vi "DAQElevador.vi"() -> ()   [LabVIEW 2018]
uses:
  EstadoElevador.ctl
panel:
  out "Piso":u32
  out "PteH":i32
  out "Estado Actual":T1
  out "Boton":u32
  in  "stop":bool
  in  "Sensor 1":bool
  in  "Sensor 2":bool
  in  "Sensor 3":bool
  in  "Sensor 4":bool
  in  "Piso 4":bool
  in  "Piso 3":bool
  in  "Piso 2":bool
  in  "Piso 1":bool
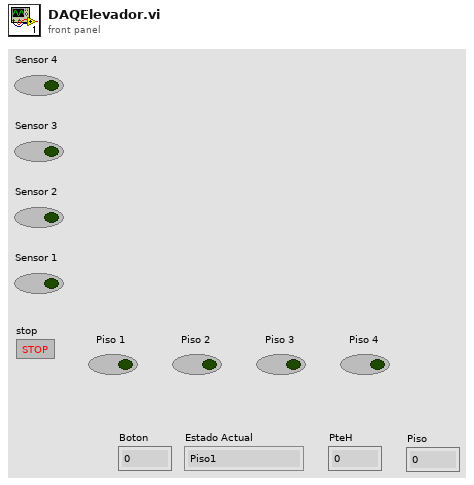
[diagram p1: front panel]
types:
  T1 = typedef "EstadoElevador.ctl" = enum16{"Piso1", "Piso2", "Piso3", "Piso4", "SubiendoPiso2", "SubiendoPiso3", "SubiendoPiso4", "BajandoPiso1", "BajandoPiso2", "BajandoPiso3"}
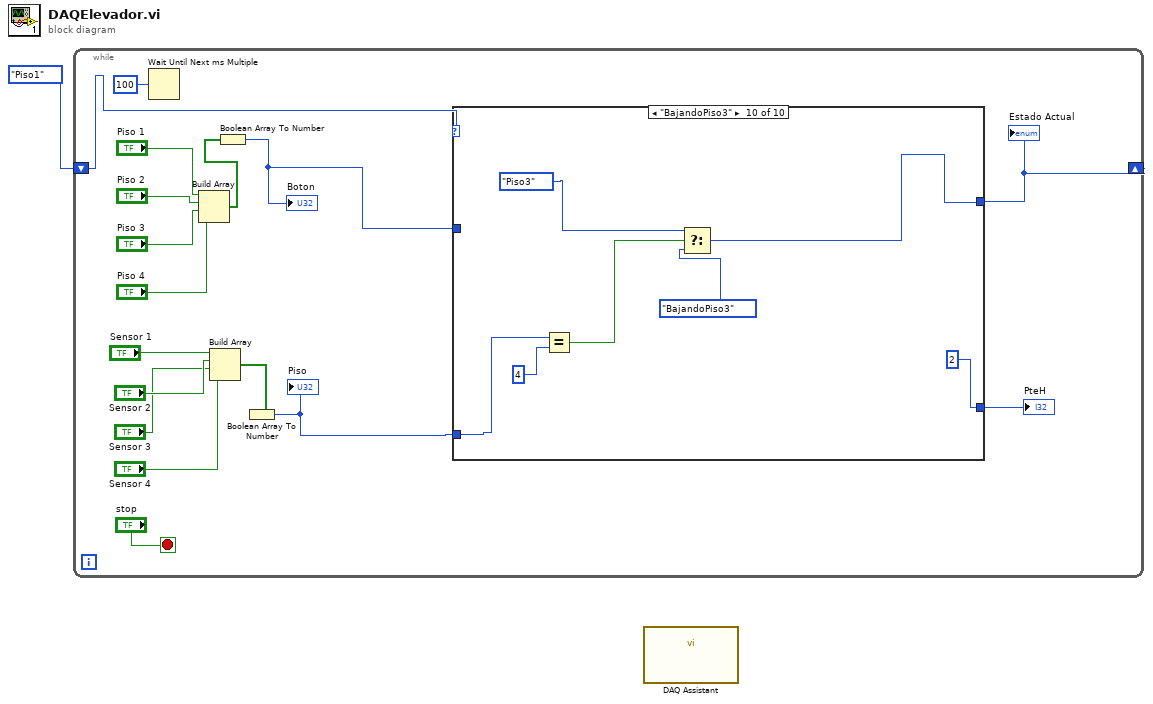
[diagram p0: block diagram]
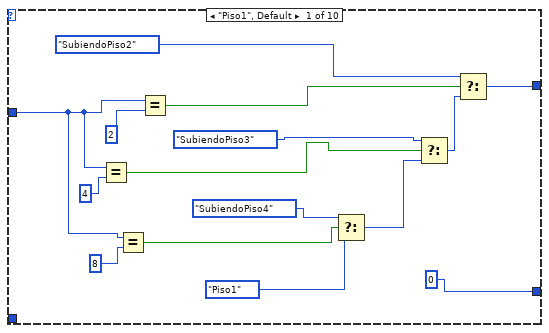
[diagram p2: hidden frame]
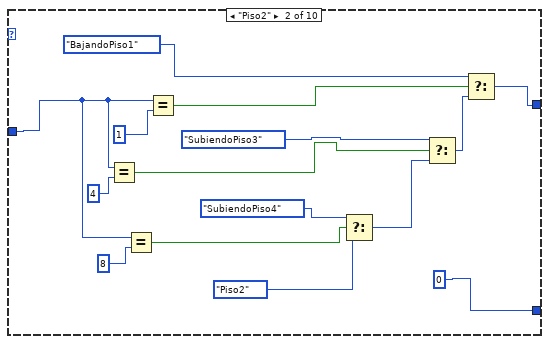
[diagram p3: hidden frame]
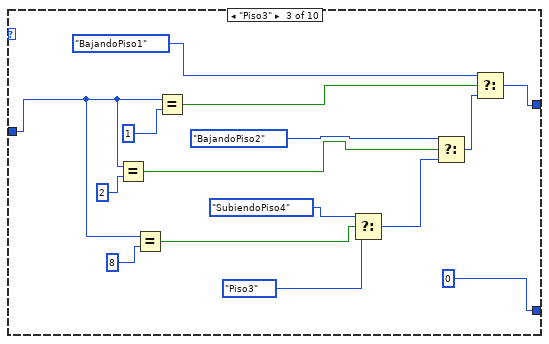
[diagram p4: hidden frame]
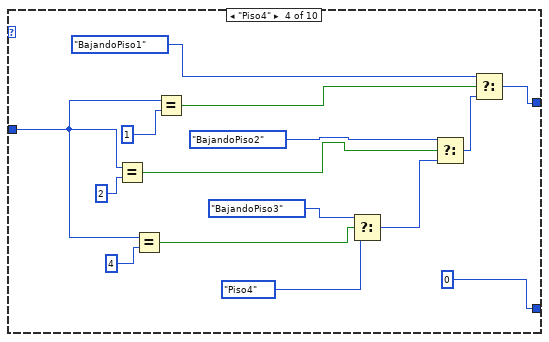
[diagram p5: hidden frame]
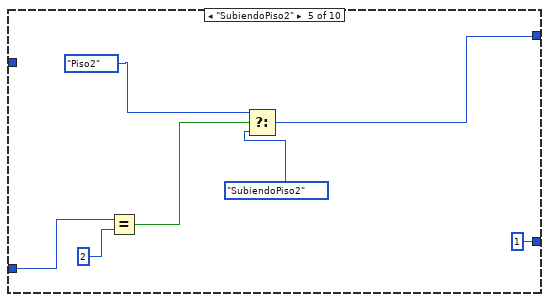
[diagram p6: hidden frame]
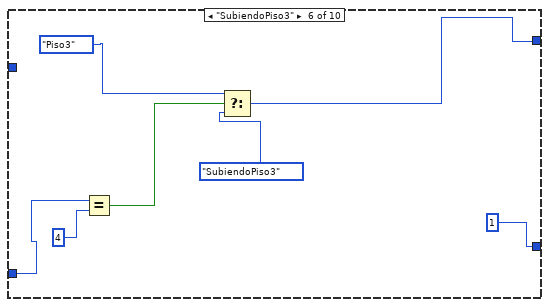
[diagram p7: hidden frame]
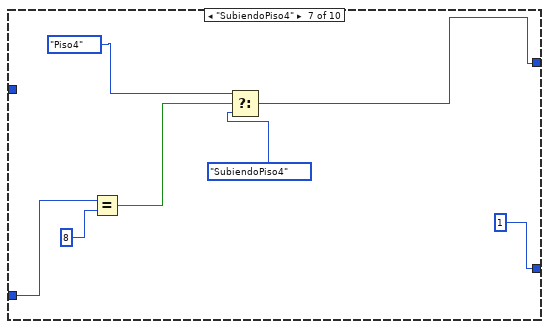
[diagram p8: hidden frame]
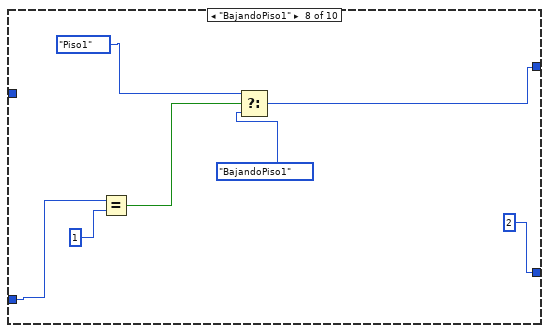
[diagram p9: hidden frame]
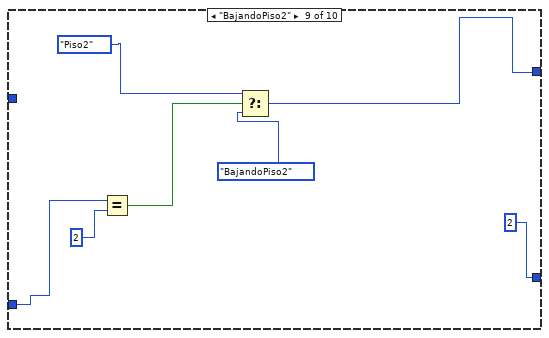
[diagram p10: hidden frame]
diagram:
  n1 = while {
    shift-right: [w14] -> _
    shift-left: EstadoElevador."Piso1" -> [w16]
    stop <- "stop" stop-if-true
    n2 = Wait Until Next ms Multiple(millisecond multiple=u32 100) -> ()  [unwired: 1 out]
    n3 = Build Array("Piso 1", "Piso 2", "Piso 3", "Piso 4") -> (w3:bool[])
    n4 = Build Array("Sensor 1", "Sensor 2", "Sensor 3", "Sensor 4") -> (w12:bool[])
    n5 = Boolean Array To Number(Boolean array=w3) -> (number=w15:u32)
    "Boton" <- w15
    n6 = Boolean Array To Number(Boolean array=w12) -> (number=w2:u32)
    "Piso" <- w2
    n7 = case shown="\"BajandoPiso3\"" w16 {
      tunnel: w15 -> [w25 w34 w49 w64 _ _ _ _ _ _]
      tunnel: [w20 w36 w50 w66 w80 w88 w95 w101 w108 w115] -> w14
      tunnel: [0 0 0 0 1 1 1 2 2 2] -> w13
      tunnel: w2 -> [_ _ _ _ w85 w87 w94 w102 w109 w116]
      frame "Piso1", Default {
        n8 = Equal?(x=w25, y=u32 4) -> (x = y?=w28:bool)
        n9 = Equal?(x=w25, y=u32 8) -> (x = y?=w24:bool)
        n10 = Equal?(x=w25, y=u32 2) -> (x = y?=w31:bool)
        n11 = Select(t=EstadoElevador."SubiendoPiso4", s=w24, f=EstadoElevador."Piso1") -> (s? t:f=w33:T1)
        n12 = Select(t=EstadoElevador."SubiendoPiso3", s=w28, f=w33) -> (s? t:f=w27:T1)
        n13 = Select(t=EstadoElevador."SubiendoPiso2", s=w31, f=w27) -> (s? t:f=w20:T1)
      }
      frame "Piso2" {
        n14 = Equal?(x=w34, y=u32 4) -> (x = y?=w46:bool)
        n15 = Equal?(x=w34, y=u32 8) -> (x = y?=w48:bool)
        n16 = Equal?(x=w34, y=u32 1) -> (x = y?=w45:bool)
        n17 = Select(t=EstadoElevador."SubiendoPiso4", s=w48, f=EstadoElevador."Piso2") -> (s? t:f=w44:T1)
        n18 = Select(t=EstadoElevador."SubiendoPiso3", s=w46, f=w44) -> (s? t:f=w47:T1)
        n19 = Select(t=EstadoElevador."BajandoPiso1", s=w45, f=w47) -> (s? t:f=w36:T1)
      }
      frame "Piso3" {
        n20 = Equal?(x=w49, y=u32 2) -> (x = y?=w61:bool)
        n21 = Equal?(x=w49, y=u32 8) -> (x = y?=w59:bool)
        n22 = Equal?(x=w49, y=u32 1) -> (x = y?=w62:bool)
        n23 = Select(t=EstadoElevador."SubiendoPiso4", s=w59, f=EstadoElevador."Piso3") -> (s? t:f=w63:T1)
        n24 = Select(t=EstadoElevador."BajandoPiso2", s=w61, f=w63) -> (s? t:f=w60:T1)
        n25 = Select(t=EstadoElevador."BajandoPiso1", s=w62, f=w60) -> (s? t:f=w50:T1)
      }
      frame "Piso4" {
        n26 = Equal?(x=w64, y=u32 2) -> (x = y?=w76:bool)
        n27 = Equal?(x=w64, y=u32 4) -> (x = y?=w74:bool)
        n28 = Equal?(x=w64, y=u32 1) -> (x = y?=w77:bool)
        n29 = Select(t=EstadoElevador."BajandoPiso3", s=w74, f=EstadoElevador."Piso4") -> (s? t:f=w78:T1)
        n30 = Select(t=EstadoElevador."BajandoPiso2", s=w76, f=w78) -> (s? t:f=w75:T1)
        n31 = Select(t=EstadoElevador."BajandoPiso1", s=w77, f=w75) -> (s? t:f=w66:T1)
      }
      frame "SubiendoPiso2" {
        n32 = Equal?(x=w85, y=u32 2) -> (x = y?=w84:bool)
        n33 = Select(t=EstadoElevador."Piso2", s=w84, f=EstadoElevador."SubiendoPiso2") -> (s? t:f=w80:T1)
      }
      frame "SubiendoPiso3" {
        n34 = Equal?(x=w87, y=u32 4) -> (x = y?=w92:bool)
        n35 = Select(t=EstadoElevador."Piso3", s=w92, f=EstadoElevador."SubiendoPiso3") -> (s? t:f=w88:T1)
      }
      frame "SubiendoPiso4" {
        n36 = Equal?(x=w94, y=u32 8) -> (x = y?=w99:bool)
        n37 = Select(t=EstadoElevador."Piso4", s=w99, f=EstadoElevador."SubiendoPiso4") -> (s? t:f=w95:T1)
      }
      frame "BajandoPiso1" {
        n38 = Equal?(x=w102, y=u32 1) -> (x = y?=w106:bool)
        n39 = Select(t=EstadoElevador."Piso1", s=w106, f=EstadoElevador."BajandoPiso1") -> (s? t:f=w101:T1)
      }
      frame "BajandoPiso2" {
        n40 = Equal?(x=w109, y=u32 2) -> (x = y?=w113:bool)
        n41 = Select(t=EstadoElevador."Piso2", s=w113, f=EstadoElevador."BajandoPiso2") -> (s? t:f=w108:T1)
      }
      frame "BajandoPiso3" {
        n42 = Equal?(x=w116, y=u32 4) -> (x = y?=w120:bool)
        n43 = Select(t=EstadoElevador."Piso3", s=w120, f=EstadoElevador."BajandoPiso3") -> (s? t:f=w115:T1)
      }
    }
    "Estado Actual" <- w14
    "PteH" <- w13
  }
  n44 = call "DAQ Assistant"() -> ()  [unwired: 12 in]
